vi "configure.vi"(8 "error in (no error)":errorcluster, 11 "DL090216RangeOffsetImageProcessor in":refnum<class "ImageProcessorDL090216RangeOffset.lvclass">) -> (0 "error out":errorcluster, 3 "DL090216RangeOffsetImageProcessor out":refnum<class "ImageProcessorDL090216RangeOffset.lvclass">)   [LabVIEW 2010, in "ImageProcessorDL090216RangeOffset.lvclass"]
uses:
  ImageProcessorDL090216RangeOffset.lvclass
  ImageProcessorDL090216RangeOffset.lvclass/ImageProcessorDL090216RangeOffset.ctl
  common/classes/GenericComponent/GenericComponent/GenericComponent.lvclass
panel:
  in  "Tab Control":enum32{"Description", "Configuration settings "}(tab)
  in  "maximum value":dbl
  out "Configuration":string
  in  "cancel":bool
  in  "save":bool
  # "Configure ImageProcessorDL090216RangeOffset"
  # "The ImageProcessorDL090216RangeOffset component adjusts range and offset of gray-scale images."
  # "This is the maximum expected image intensity value."
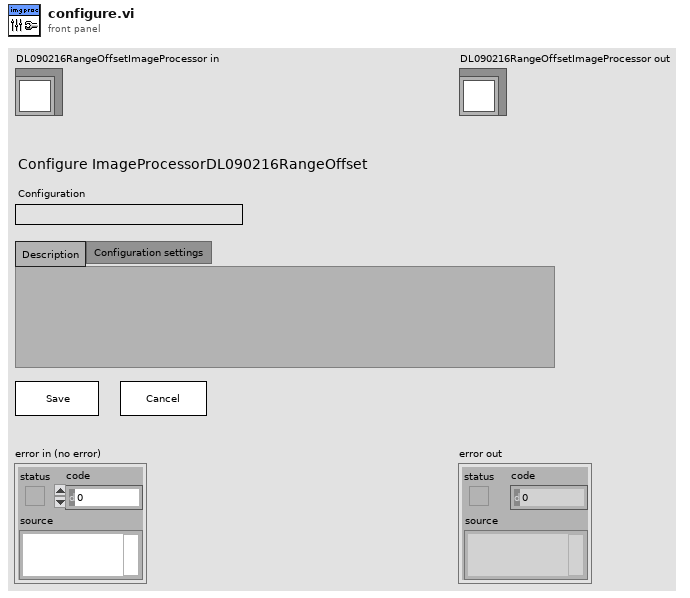
[diagram p1: front panel]
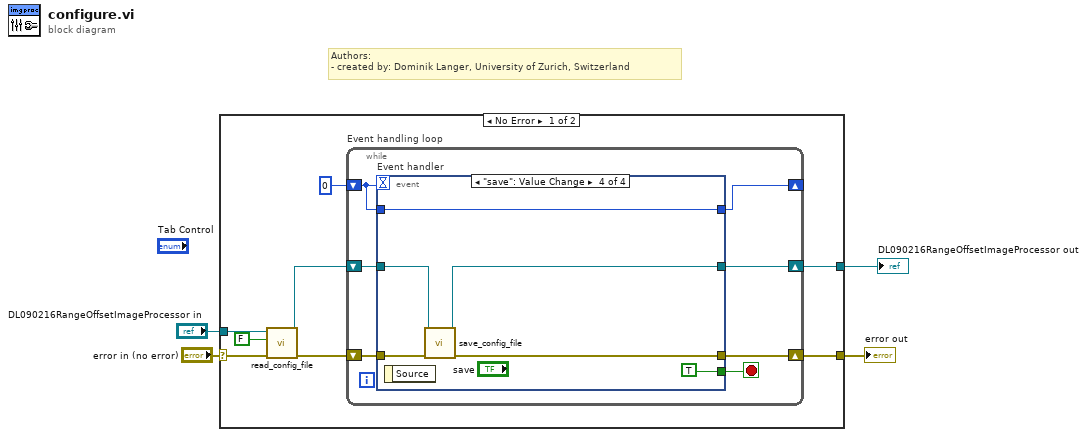
[diagram p0: block diagram]
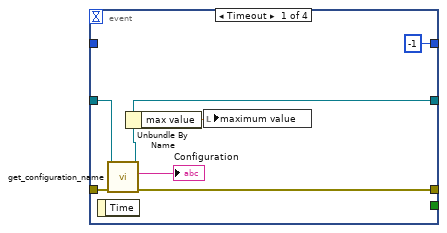
[diagram p2: hidden frame]
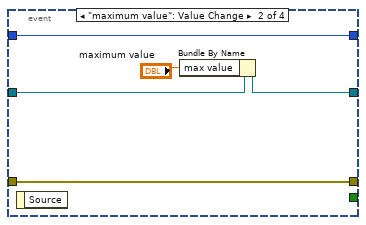
[diagram p3: hidden frame]
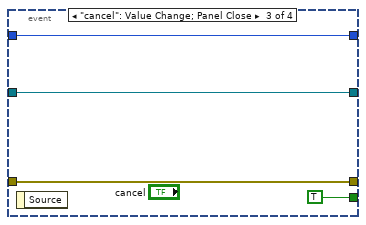
[diagram p4: hidden frame]
diagram:
  # "Authors: \n- created by: Dominik Langer, University of Zurich, Switzerland"
  n1 = case shown="No Error" "error in (no error)" {
    selector: "error in (no error)" -> [w12 w43]
    tunnel: [w5 w43] -> w3
    tunnel: [w6 w42] -> w1
    tunnel: "DL090216RangeOffsetImageProcessor in" -> [w10 w42]
    frame No Error {
      n2 = call-dynamic "read_config_file.vi"("error in (no error)"=w12, "force load?"=FALSE, "GenericPlugin in"=w10) -> ("error out"=w8:errorcluster, "GenericPlugin out"=w9:refnum<class "ImageProcessorDL090216RangeOffset.lvclass">)  [unwired: 7 out]
      n3 = while "Event handling loop" {
        shift-right: [w16] -> w6
        shift-left: w9 -> [w17]
        shift-right: [w18] -> w5
        shift-left: w8 -> [w19]
        shift-right: [w14] -> _
        shift-left: 0 -> [w15]
        stop <- w13 stop-if-true
        n4 = event "Event handler" shown="[3] \"save\": Value Change" {
          selector: _ -> [_ _ _ _]
          dyn-events: _ -> [_ _ _ _]
          timeout: w15 -> [_ _ _ _]
          tunnel: [w23 w31 w35 w39] -> w18
          tunnel: w19 -> [w24 w31 w35 w40]
          tunnel: w17 -> [w22 w30 w32 w36]
          tunnel: [w21 w29 w32 w38] -> w16
          tunnel: [-1 w27 w34 w41] -> w14
          tunnel: w15 -> [_ w27 w34 w41]
          tunnel: [_ _ TRUE TRUE] -> w13
          event Timeout {
            n5 = event-data() -> ()  [unwired: 2 out]
            n6 = call "get_configuration_name.vi"("error in (no error)"=w24, "GenericPlugin.lvclass in"=w22) -> ("error out"=w23:errorcluster, "configuration name"=→"Configuration":string, "GenericPlugin.lvclass out"=w21:refnum<class "ImageProcessorDL090216RangeOffset.lvclass">)  [unwired: 7 in]
            n7 = Unbundle By Name(w21) -> ("max value"=w25:dbl)
            n8 = local write "maximum value"(w25) -> ()
          }
          event "maximum value": Value Change {
            n9 = event-data() -> ()  [unwired: 2 out]
            n10 = Bundle By Name(cluster=w30, "max value"="maximum value") -> (w29:refnum<class "ImageProcessorDL090216RangeOffset.lvclass">)
          }
          event "cancel": Value Change; Panel Close {
            n11 = event-data() -> ()  [unwired: 2 out]
          }
          event "save": Value Change {
            n12 = event-data() -> ()  [unwired: 2 out]
            n13 = call-dynamic "save_config_file.vi"("error in (no error)"=w40, "GenericPlugin in"=w36) -> ("error out"=w39:errorcluster, "GenericPlugin out"=w38:refnum<class "ImageProcessorDL090216RangeOffset.lvclass">)  [unwired: 2 in, 6 out]
          }
        }
      }
    }
    frame Error {
    }
  }
  "error out" <- w3
  "DL090216RangeOffsetImageProcessor out" <- w1
